vi "Protocol.vi"(0 "FC":enum16{"读", "单个配置", "多个配置"}(ring) caption="功能码", 1 "mAdr":u8=1 caption="从设备地址" min=1 max=250 format="%x", 7 "regAdr":u16=1 caption="起始寄存器地址" format="%x", 11 "num":u16=1 caption="寄存器个数/数值", 12 "values":string) -> (6 "dtStr":string, 10 "rdMatch":string)   [LabVIEW 2015]
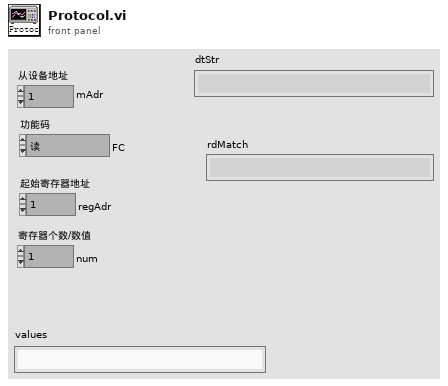
[diagram p1: front panel]
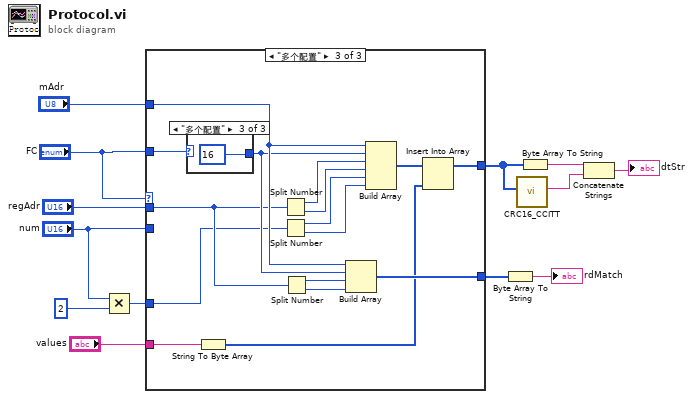
[diagram p0: block diagram]
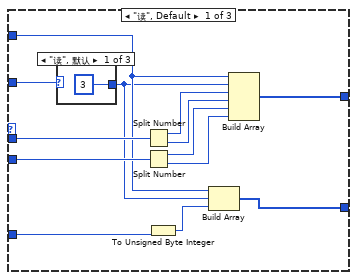
[diagram p2: hidden frame]
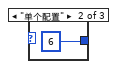
[diagram p3: hidden frame]
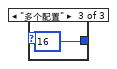
[diagram p4: hidden frame]
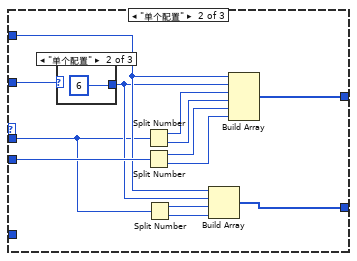
[diagram p5: hidden frame]
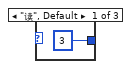
[diagram p6: hidden frame]
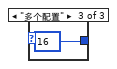
[diagram p7: hidden frame]
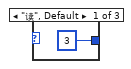
[diagram p8: hidden frame]
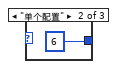
[diagram p9: hidden frame]
diagram:
  n1 = Multiply(x="num", y=u16 2) -> (x*y=w3:u16)
  n2 = case shown="\"多个配置\"" "FC" {
    tunnel: "FC" -> [w26 w42 w61]
    tunnel: "regAdr" -> [w25 w32 w53]
    tunnel: [w20 w37 w48] -> w12
    tunnel: "num" -> [w19 w36 _]
    tunnel: "mAdr" -> [w18 w35 w56]
    tunnel: [w16 w33 w54] -> w5
    tunnel: w3 -> [w15 _ w50]
    tunnel: "values" -> [_ _ w47]
    frame "读", Default {
      n3 = case shown="\"读\", 默认" w26 {
        tunnel: [u8 3 ("mAdr") u8 6 ("mAdr") u8 16 ("mAdr")] -> w17
        frame "读", Default {
        }
        frame "单个配置" {
        }
        frame "多个配置" {
        }
      }
      n4 = Split Number(x=w25) -> (hi(x)=w24:u8, lo(x)=w23:u8)
      n5 = Split Number(x=w19) -> (hi(x)=w22:u8, lo(x)=w21:u8)
      n6 = To Unsigned Byte Integer(number=w15) -> (unsigned 8bit integer=w14:u8)
      n7 = Build Array(w18, w17, w14) -> (w16:u8[])
      n8 = Build Array(w18, w17, w24, w23, w22, w21) -> (w20:u8[])
    }
    frame "单个配置" {
      n9 = case shown="\"单个配置\"" w42 {
        tunnel: [u8 3 ("mAdr") u8 6 ("mAdr") u8 16 ("mAdr")] -> w34
        frame "读", Default {
        }
        frame "单个配置" {
        }
        frame "多个配置" {
        }
      }
      n10 = Split Number(x=w32) -> (hi(x)=w41:u8, lo(x)=w40:u8)
      n11 = Split Number(x=w36) -> (hi(x)=w39:u8, lo(x)=w38:u8)
      n12 = Split Number(x=w32) -> (hi(x)=w31:u8, lo(x)=w30:u8)
      n13 = Build Array(w35, w34, w31, w30) -> (w33:u8[])
      n14 = Build Array(w35, w34, w41, w40, w39, w38) -> (w37:u8[])
    }
    frame "多个配置" {
      n15 = case shown="\"多个配置\"" w61 {
        tunnel: [u8 3 ("mAdr") u8 6 ("mAdr") u8 16 ("mAdr")] -> w55
        frame "读", Default {
        }
        frame "单个配置" {
        }
        frame "多个配置" {
        }
      }
      n16 = String To Byte Array(string=w47) -> (unsigned byte array=w46:u8[])
      n17 = Split Number(x=w53) -> (hi(x)=w60:u8, lo(x)=w59:u8)
      n18 = Split Number(x=w50) -> (hi(x)=w58:u8, lo(x)=w57:u8)
      n19 = Split Number(x=w53) -> (hi(x)=w52:u8, lo(x)=w51:u8)
      n20 = Build Array(w56, w55, w52, w51) -> (w54:u8[])
      n21 = Build Array(w56, w55, w60, w59, w58, w57) -> (w49:u8[])
      n22 = Insert Into Array(array=w49, new element=w46) -> (w48:u8[])  [unwired: 1 in]
    }
  }
  n23 = Byte Array To String(unsigned byte array=w5) -> (string=→"rdMatch":string)
  n24 = call "CRC16_CCITT.vi"("iDt"=w12) -> ("CRC16_LH"=w10:string)  [unwired: 8 in, 2 out]
  n25 = Byte Array To String(unsigned byte array=w12) -> (string=w11:string)
  n26 = Concatenate Strings(w11, w10) -> (→"dtStr":string)
